vi "CLD 15 Address Parsing SubVI.vi"(8 "error in":errorcluster, 10 "Data String in":string, 11 "CSV File Data Structure in":T1) -> (0 "error out":errorcluster, 3 "CSV File Data Structure out":T1)   [LabVIEW 2009]
doc: "CLD 15 Parsing routine for the address sting in CLD 15. This String also includes the price discount as a percent. The values of the price and large order threshold are taken from the specification.\n\nThe data formats are copied as free labels from the specification to avoid re-checking the specification during programming."
uses:
  CLD 15 CSV file data structure.ctl
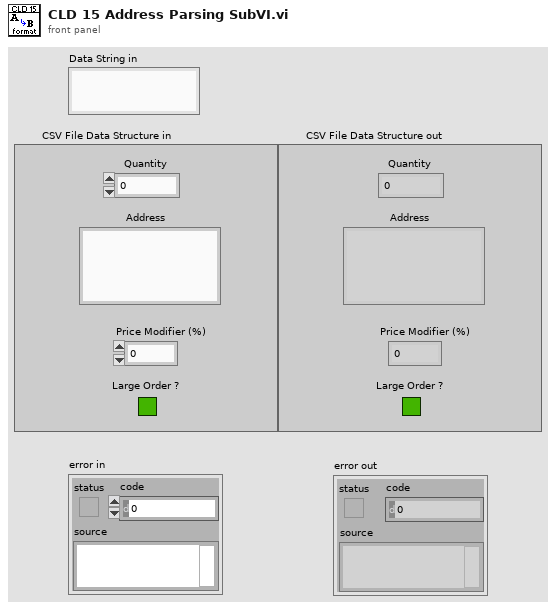
[diagram p1: front panel]
types:
  T1 = typedef "CLD 15 CSV file data structure.ctl" = cluster{"Quantity":i32, "Address":string, "Price Modifier (%)":dbl, "Large Order ?":bool}
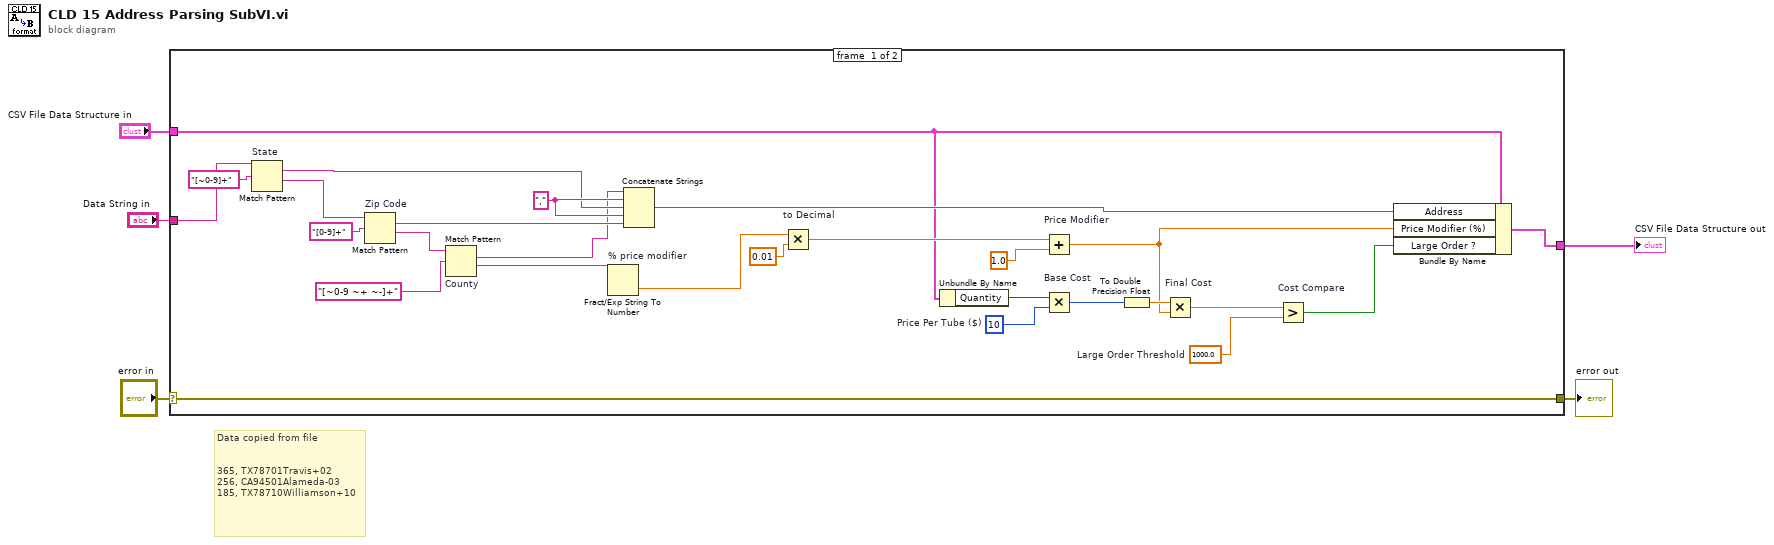
[diagram p0: block diagram]
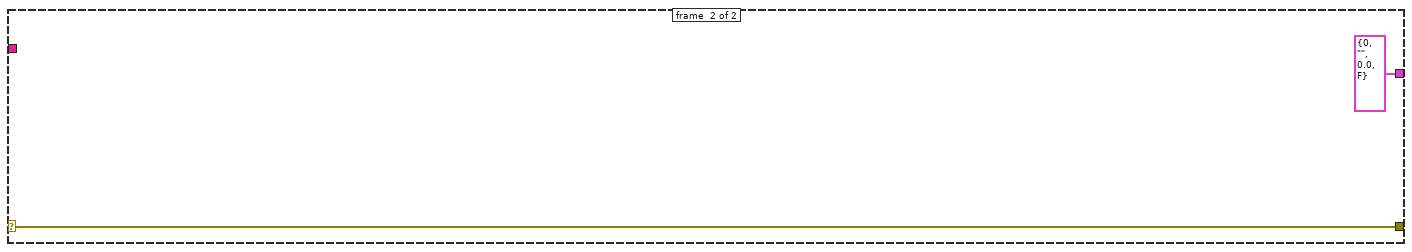
[diagram p2: hidden frame]
diagram:
  # "Data copied from file\n\n\n365,\tTX78701Travis+02\n256,\tCA94501Alameda-03\n185,\tTX78710Williamson+10"
  n1 = case shown="No Error" "error in" {
    selector: "error in" -> [w7 w34]
    tunnel: [w32 T1 {"Quantity"=0, "Address"="", "Price Modifier (%)"=0.0, "Large Order ?"=FALSE} ("CSV File Data Structure in")] -> w5
    tunnel: "Data String in" -> [w31 _]
    tunnel: [w7 w34] -> w2
    tunnel: "CSV File Data Structure in" -> [w6 _]
    frame #0 {
      w14 = 1000.0  # Large Order Threshold
      w19 = 10  # Price Per Tube ($)
      w29 = ","
      n2 = Match Pattern "State"(string=w31, regular expression="[~0-9]+") -> (match substring=w28:string, after substring=w27:string)  [unwired: 1 in, 2 out]
      n3 = Match Pattern "Zip Code"(string=w27, regular expression="[0-9]+") -> (match substring=w25:string, after substring=w24:string)  [unwired: 1 in, 2 out]
      n4 = Match Pattern "County"(string=w24, regular expression="[~0-9 ~+ ~-]+") -> (match substring=w23:string, after substring=w21:string)  [unwired: 1 in, 2 out]
      n5 = Fract/Exp String To Number "% price modifier"(string=w21) -> (number=w9:dbl)  [unwired: 3 in, 1 out]
      n6 = Concatenate Strings(w23, w29, w28, w29, w25) -> (w22:string)
      n7 = Multiply "to Decimal"(x=w9, y=0.01) -> (x*y=w8:dbl)
      n8 = Unbundle By Name(w6) -> ("Quantity"=w20:i32)
      n9 = Add "Price Modifier"(x=w8, y=1.0) -> (x+y=w11:dbl)
      n10 = Multiply "Base Cost"(x=w20, y=w19) -> (x*y=w17:i32)
      n11 = To Double Precision Float(number=w17) -> (double precision float=w16:dbl)
      n12 = Multiply "Final Cost"(x=w16, y=w11) -> (x*y=w15:dbl)
      n13 = Greater? "Cost Compare"(x=w15, y=w14) -> (0:w13:bool)
      n14 = Bundle By Name(cluster=w6, "Address"=w22, "Price Modifier (%)"=w11, "Large Order ?"=w13) -> (w32:T1)
    }
    frame #1 {
    }
  }
  "CSV File Data Structure out" <- w5
  "error out" <- w2
